vi "BoolArray to UINT8Array.vi"(1 "Input Array (Bool)":bool[](array[boolean])) -> (0 "Output Array (UINT_8)":u8[](array[numeric]))   [LabVIEW 2014]
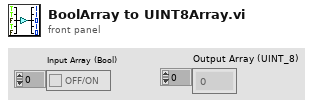
[diagram p1: front panel]
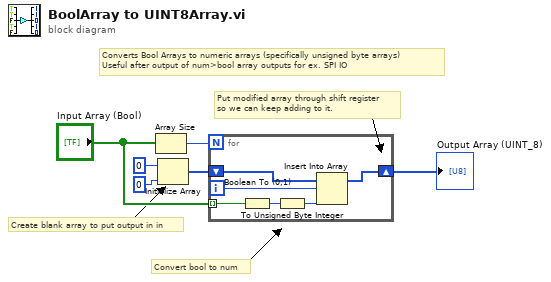
[diagram p0: block diagram]
diagram:
  # "Put modified array through shift register\nso we can keep adding to it."
  # "Convert bool to num"
  # "Create blank array to put output in in"
  # "Converts Bool Arrays to numeric arrays (specifically unsigned byte arrays)\nUseful after output of num>bool array outputs for ex. SPI IO"
  n1 = Array Size(array="Input Array (Bool)") -> (size(s)=w5:i32)
  n2 = Initialize Array(u8 0, 0) -> (w4:u8[])
  n3 = for {
    N: w5 -> [_]
    tunnel: "Input Array (Bool)" -> [w12] mode=indexing
    shift-right: [w9] -> w2
    shift-left: w4 -> [w10]
    i -> [w11]
    n4 = Boolean To (0,1)(Boolean=w12) -> (0, 1=w8:i16)
    n5 = To Unsigned Byte Integer(number=w8) -> (unsigned 8bit integer=w7:u8)
    n6 = Insert Into Array(array=w10, index=w11, new element=w7) -> (w9:u8[])
  }
  "Output Array (UINT_8)" <- w2
